vi "Curtin1_updatePlots.vi"(9 "plots":refnum<vi>[](array[refnum]), 11 "Settings":T1={"Name of test"="ScratchPad", "Date"=timestamp(0 s since 1904-01-01), "Location"="Home", "Template"="ScratchPad", "Soundcard"="OCTA-CAPTURE", "resolution"=32, "Sampling rate"=48000, "Ch1 Gain "=25.0, "Ch2 Gain"=10.0, "Sample time (s)"=0.3, "Pre-trigger (s)"=0.001, "Hammer Threshold"=0.021311, "Positions"=12, "Taps/Position"=5, "Set Names"="H,V", "Freq resolution"=1.0, "Hammer cutoff"=0.025, "Mic cutoff"=0.25, "Double bounce "=0.01, "Hammer Cal"=1.0, "dB Offset"=0.0, "Accel Cal"=10.0, "Vibrometer Cal"=1.0, "Mic Cal"=1.0, "Output"=2, "Voltage Cal"=1.0, "Vibrometer Port"="ASRL27::INSTR", "Range"=4, "High Pass"=2, "Bandwidth"=4, "X Range"=[{"Minimum"=200.0, "Maximum"=10000.0, "Increment"=10.0, "Minor Increment"=100.0, "Start"=200.0}, {"Minimum"=0.0, "Maximum"=0.05, "Increment"=0.025, "Minor Increment"=0.0025, "Start"=0.0}, {"Minimum"=0.0, "Maximum"=0.3, "Increment"=0.1, "Minor Increment"=0.01, "Start"=0.0}, {"Minimum"=200.0, "Maximum"=10000.0, "Increment"=10.0, "Minor Increment"=100.0, "Start"=1000.0}], "Y Range"=[{"Minimum"=-25.0, "Maximum"=0.0, "Increment"=5.0, "Minor Increment"=1.0, "Start"=-25.0}, {"Minimum"=-0.1, "Maximum"=0.1, "Increment"=0.05, "Minor Increment"=0.01, "Start"=-0.1}, {"Minimum"=-0.1, "Maximum"=0.1, "Increment"=0.05, "Minor Increment"=0.01, "Start"=-0.1}, {"Minimum"=-20.0, "Maximum"=20.0, "Increment"=2.0, "Minor Increment"=0.5, "Start"=-20.0}], "dB Spread"=40.0, "Trigger"=0, "Ch_1"=1, "Ch_2"=2, "flip?"=FALSE, "60Hz"=FALSE, "Time offset"=0.0, "Piezo Cal"=1.0, "Default Notes"=""} {"Ch_2" min=1 step=1; "Ch_1" min=1 max=100 step=1; "Trigger" items=["Hammer (force)", "Self-tap", "Spacebar"]; "Bandwidth" items=["1 kHz"=1, "5 kHz"=5, "10 kHz"=10, "25 kHz"=25, "50 kHz"=50, "100 kHz"=100]; "High Pass" items=["Off", "13 Hz", "104 Hz"]; "Range" items=["10 mm/s"=1, "20 mm/s"=2, "50 mm/s"=5, "100 mm/s"=10, "200 mm/s"=20, "500 mm/s"=50, "1 m/s"=100, "2 m/s"=200]; "Output" items=["Accelerometer", "Speed (from acceleration)", "Microphone", "Vibrometer", "Piezo"]; "Voltage Cal" format="%#_13g"; "Ch2 Gain" format="%#_13g"; "Ch1 Gain" format="%#_13g"; "Double bounce" min=0.0; "Mic cutoff" min=0.0 format="%#_4g"; "Hammer cutoff" min=0.0 format="%#_4g"; "Freq resolution" min=0.0; "Pre-trigger (s)" format="%#_13g"; "Date" format="%<%H:%M\n%d/%m/%y>T"; "resolution" items=["16 bit"=16, "24 bit"=24, "32 bit"=32]; "Sampling rate" items=["22050 samp/s"=22050, "44100 samp/s"=44100, "48000 samp/s"=48000]}) -> ()   [LabVIEW 2022 SP3]
uses:
  PreferencesControl.ctl
panel:
  out "output":string
  out "input":string
  # "Hz"
  # "dB"
  # "dB"
  # "sec"
  # "sec"
  # "mV/Pa"
  # "mV/m/s2"
  # "mV/mm/s"
  # "V/N"
  # "sec"
  # "sec"
  # "mV/N"
  # "a.u."
  # "a.u."
  # "sec"
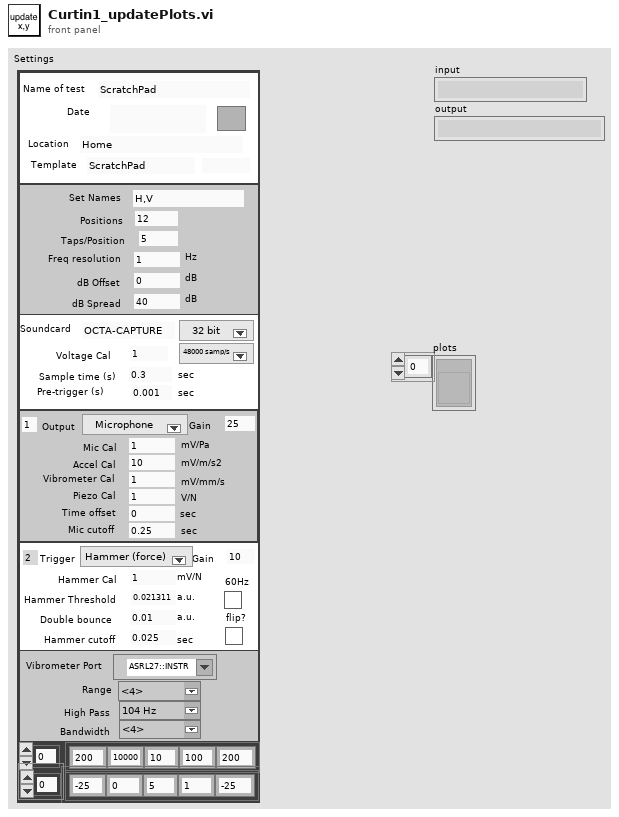
[diagram p1: front panel]
types:
  T1 = typedef "PreferencesControl.ctl" = cluster{"Name of test":string, "Date":timestamp, "Location":string, "Template":string, "Soundcard":string, "resolution":u16, "Sampling rate":u16, "Ch1 Gain ":dbl, "Ch2 Gain":dbl, "Sample time (s)":dbl, "Pre-trigger (s)":dbl, "Hammer Threshold":dbl, "Positions":i16, "Taps/Position":i16, "Set Names":string, "Freq resolution":dbl, "Hammer cutoff":dbl, "Mic cutoff":dbl, "Double bounce ":dbl, "Hammer Cal":dbl, "dB Offset":dbl, "Accel Cal":dbl, "Vibrometer Cal":dbl, "Mic Cal":dbl, "Output":u16, "Voltage Cal":dbl, "Vibrometer Port":refnum<visa-resource-name>, "Range":u16, "High Pass":u16, "Bandwidth":u16, "X Range":cluster{"Minimum":dbl, "Maximum":dbl, "Increment":dbl, "Minor Increment":dbl, "Start":dbl}[], "Y Range":cluster{"Minimum":dbl, "Maximum":dbl, "Increment":dbl, "Minor Increment":dbl, "Start":dbl}[], "dB Spread":dbl, "Trigger":u16, "Ch_1":u8, "Ch_2":u8, "flip?":bool, "60Hz":bool, "Time offset":dbl, "Piezo Cal":dbl, "Default Notes":string}
  T2 = enum16{"Acclerometer", "Displacement", "Microphone", "Vibrometer"}
  T3 = cluster{"Minimum":dbl, "Maximum":dbl, "Increment":dbl, "Minor Increment":dbl, "Start":dbl}[]
  T4 = enum8{"Enabled", "Disabled", "Disabled and Grayed Out"}
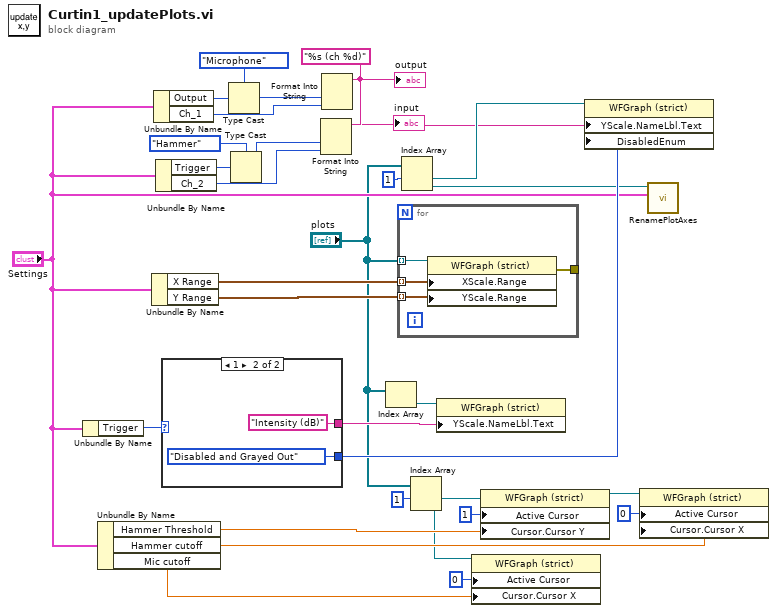
[diagram p0: block diagram]
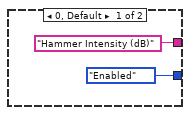
[diagram p2: hidden frame]
diagram:
  w21 = "%s (ch %d)" ("format string")
  n1 = Unbundle By Name("Settings") -> ("Trigger"=w16:u16)
  n2 = Unbundle By Name("Settings") -> ("Hammer Threshold"=w7:dbl, "Hammer cutoff"=w4:dbl, "Mic cutoff"=w1:dbl)
  n3 = Unbundle By Name("Settings") -> ("X Range"=w31:T3, "Y Range"=w30:T3)
  n4 = Unbundle By Name("Settings") -> ("Output"=w27:u16, "Ch_1"=w26:u8)
  n5 = Unbundle By Name("Settings") -> ("Trigger"=w24:u16, "Ch_2"=w25:u8)
  n6 = case shown="1" w16 {
    tunnel: ["Hammer Intensity (dB)" ("format string") "Intensity (dB)" ("format string")] -> w15
    tunnel: [T4."Enabled" ("Disabled") T4."Disabled and Grayed Out" ("Disabled")] -> w14
    frame 0, Default {
    }
    frame 1 {
    }
  }
  n7 = Type Cast(type=T2."Microphone" ("Output"), x=w27) -> (*(type *) &x=w28:T2)
  n8 = Type Cast(type=enum16{"Hammer", "Self-tap"}."Hammer" ("Input"), x=w24) -> (*(type *) &x=w23:enum16{"Hammer", "Self-tap"})
  n9 = Format Into String(format string=w21, w23, w25) -> (resulting string=w18:string)  [unwired: 2 in, 1 out]
  "input" <- w18
  n10 = Format Into String(format string=w21, w28, w26) -> (resulting string=→"output":string)  [unwired: 2 in, 1 out]
  n11 = Index Array(array="plots") -> (element=w17:refnum<vi>)  [unwired: 1 in]
  n12 = for {
    tunnel: "plots" -> [w40] mode=indexing
    tunnel: w31 -> [w39] mode=indexing
    tunnel: w30 -> [w38] mode=indexing
    tunnel: [w37] -> _
    n13 = property class="WFGraph (strict)"(reference=w40, "XScale.Range"=w39, "YScale.Range"=w38) -> (error out=w37:errorcluster)  [unwired: 1 in, 1 out]
  }
  n14 = Index Array(array="plots", index #1=1 ("index")) -> (element #1=w20:refnum<vi>, element #2=w13:refnum<vi>)  [unwired: 1 in]
  n15 = Index Array(array="plots", index #1=1 ("index")) -> (element #1=w9:refnum<vi>, element #2=w2:refnum<vi>)  [unwired: 1 in]
  n16 = property class="WFGraph (strict)"(reference=w17, "YScale.NameLbl.Text"=w15) -> ()  [unwired: 1 in, 2 out]
  n17 = property class="WFGraph (strict)"(reference=w2, "Active Cursor"=u32 0, "Cursor.Cursor X"=w1) -> ()  [unwired: 1 in, 2 out]
  n18 = property class="WFGraph (strict)"(reference=w9, "Active Cursor"=u32 1, "Cursor.Cursor Y"=w7) -> (reference out=w5:refnum<vi>)  [unwired: 1 in, 1 out]
  n19 = property class="WFGraph (strict)"(reference=w20, "YScale.NameLbl.Text"=w18, "DisabledEnum"=w14) -> ()  [unwired: 1 in, 2 out]
  n20 = property class="WFGraph (strict)"(reference=w5, "Active Cursor"=u32 0, "Cursor.Cursor X"=w4) -> ()  [unwired: 1 in, 2 out]
  n21 = call "RenamePlotAxes.vi"("Settings"="Settings", "WaveformGraph in"=w13) -> ()  [unwired: 10 in]
